vi "BatteryWarningTest_3.2V.vi"(8 "error in":errorcluster) -> (0 "error in (no error)":errorcluster, 1 "Pass/Fail":bool, 4 "Limit2":u8[](array[numeric]) format="%x", 5 "Limit1":u8[](array[numeric]) format="%x")   [LabVIEW 2009]
uses:
  <vilib>/Instr/_visa.llb/VISA Configure Serial Port (Instr).vi
  Global/Global 1.vi
panel:
  # "30"
  # "0A"
  # "0A"
  # "31"
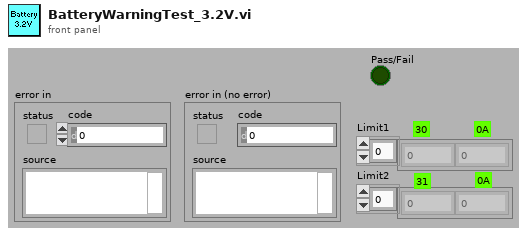
[diagram p1: front panel]
types:
  T1 = cluster{"VHEATFUSENOLOADMIN":string, "VHEATFUSELOADMAX":string, "VOVERRIDEDIODEMIN":string, "TDIFFMAX":string, "MEASFREQMAX":string, "MEASFREQMIN":string, "VOVER":string, "VMIDDLE":string, "VUNDER":string, "VNORESET":string, "VRESET":string, "WAITPING":string, "LRFID":string, "RFIDUID":string, "EXTEESIZE":string, "LCUTYPE":string, "LCUSUBTYPE":string, "TEVN":string, "BOOTVER":string, "APPVER":string, "ISLEEPMAX":string, "TSLEEP":string, "APPWAIT":string, "DBWAIT":string}
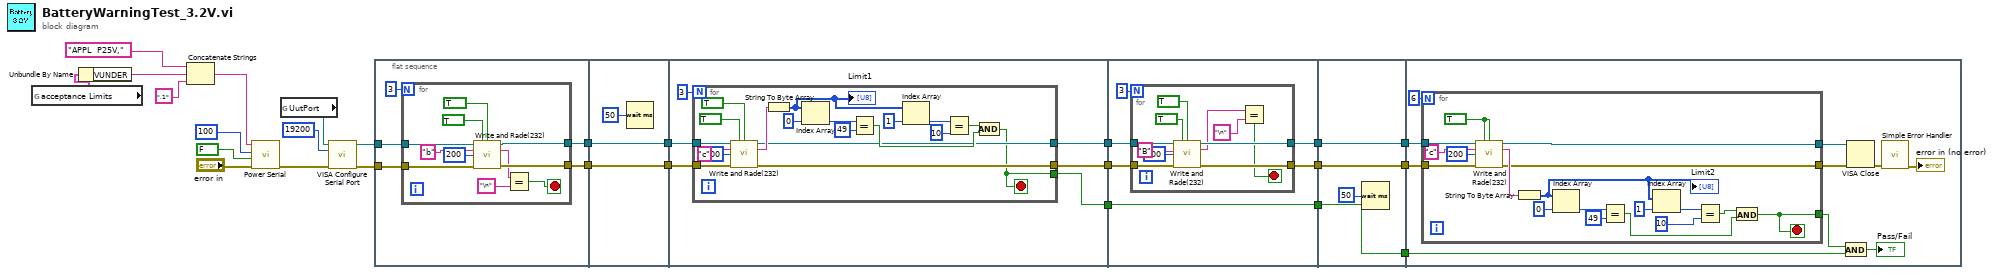
[diagram p0: block diagram]
diagram:
  n1 = global read "Global 1.vi" "acceptance Limits"() -> (w5:T1)
  n2 = Unbundle By Name(w5) -> ("VUNDER"=w4:string)
  n3 = Concatenate Strings("APPL  P25V," ("In"), w4, ",1" ("string")) -> (w1:string)
  n4 = call "Power Serial.vi"("error in (no error)"="error in", "Rd?"=FALSE, "Delay"=100, "IN"=w1) -> ("error out"=w11:errorcluster)  [unwired: 1 in, 6 out]
  n5 = global read "Global 1.vi" "UutPort"() -> (w12:refnum<visa-resource-name>)
  n6 = call-poly "VISA Configure Serial Port"("VISA resource name"=w12, "baud rate (9600)"=u32 19200, "error in (no error)"=w11) -> ("VISA resource name out"=w6:refnum<visa-resource-name>, "error out"=w7:errorcluster)  [unwired: 3 in, 8 out]
  n7 = flat-sequence {
    tunnel: [w31] -> w23
    tunnel: [w30] -> w21
    tunnel: w7 -> [w28]
    tunnel: w6 -> [w27]
    tunnel: w23 -> [w44]
    tunnel: [w44] -> w22
    tunnel: w21 -> [w43]
    tunnel: [w43] -> w20
    tunnel: [w51] -> w24
    tunnel: w22 -> [w50]
    tunnel: w20 -> [w49]
    tunnel: [w48] -> w19
    tunnel: [w47] -> w18
    tunnel: [w76] -> w25
    tunnel: w24 -> [w76]
    tunnel: w19 -> [w75]
    tunnel: w18 -> [w74]
    tunnel: [w73] -> w17
    tunnel: [w72] -> w15
    tunnel: [w90] -> w26
    tunnel: w25 -> [w90]
    tunnel: w17 -> [w89]
    tunnel: [w89] -> w16
    tunnel: w15 -> [w88]
    tunnel: [w88] -> w14
    tunnel: w26 -> [w101]
    tunnel: w16 -> [w98]
    tunnel: w14 -> [w97]
    frame #0 {
      n8 = for {
        N: 3 -> [_]
        tunnel: w28 -> [w41]
        tunnel: w27 -> [w40]
        tunnel: [w39] -> w31
        tunnel: [w38] -> w30
        stop <- w33 stop-if-true
        n9 = call "Write and Rade(232).vi"("VISA resource name in"=w40, "write"=TRUE, "read"=TRUE, "string to write"="b", "ms delay"=u32 200, "error in"=w41) -> ("VISA resource name out"=w39:refnum<visa-resource-name>, "read string"=w35:string, "error out"=w38:errorcluster)  [unwired: 2 in, 5 out]
        n10 = Equal?(x=w35, y="\n") -> (x = y?=w33:bool)
      }
    }
    frame #1 {
      n11 = Wait (ms)(milliseconds to wait=u32 50) -> ()  [unwired: 1 out]
    }
    frame #2 {
      n12 = for {
        N: 3 -> [_]
        tunnel: [w53] -> w51
        tunnel: w50 -> [w60]
        tunnel: w49 -> [w59]
        tunnel: [w55] -> w48
        tunnel: [w54] -> w47
        stop <- w53 stop-if-true
        n13 = call "Write and Rade(232).vi"("VISA resource name in"=w60, "write"=TRUE, "read"=TRUE, "string to write"="c", "ms delay"=u32 200, "error in"=w59) -> ("VISA resource name out"=w54:refnum<visa-resource-name>, "read string"=w56:string, "error out"=w55:errorcluster)  [unwired: 2 in, 5 out]
        n14 = String To Byte Array(string=w56) -> (unsigned byte array=w65:u8[])
        "Limit1" <- w65
        n15 = Index Array(array=w65, index=0) -> (element=w63:u8)
        n16 = Equal?(x=w63, y=u8 49) -> (x = y?=w70:bool)
        n17 = Index Array(array=w65, index=1) -> (element=w67:u8)
        n18 = Equal?(x=w67, y=u8 10) -> (x = y?=w69:bool)
        n19 = And(x=w69, y=w70) -> (x .and. y?=w53:bool)
      }
    }
    frame #3 {
      n20 = for {
        N: 3 -> [_]
        tunnel: w75 -> [w87]
        tunnel: w74 -> [w85]
        tunnel: [w84] -> w73
        tunnel: [w83] -> w72
        stop <- w78 stop-if-true
        n21 = call "Write and Rade(232).vi"("VISA resource name in"=w85, "write"=TRUE, "read"=TRUE, "string to write"="B", "ms delay"=u32 200, "error in"=w87) -> ("VISA resource name out"=w83:refnum<visa-resource-name>, "read string"=w80:string, "error out"=w84:errorcluster)  [unwired: 2 in, 5 out]
        n22 = Equal?(x=w80, y="\n") -> (x = y?=w78:bool)
      }
    }
    frame #4 {
      n23 = Wait (ms)(milliseconds to wait=u32 50) -> ()  [unwired: 1 out]
    }
    frame #5 {
      n24 = for {
        N: 6 -> [_]
        tunnel: [w103] -> w99
        tunnel: w98 -> [w109]
        tunnel: w97 -> [w108]
        tunnel: [w106] -> w96
        tunnel: [w105] -> w94
        stop <- w103 stop-if-true
        w104 = TRUE ("write")
        n25 = call "Write and Rade(232).vi"("VISA resource name in"=w108, "write"=w104, "read"=w104, "string to write"="c", "ms delay"=u32 200, "error in"=w109) -> ("VISA resource name out"=w105:refnum<visa-resource-name>, "read string"=w107:string, "error out"=w106:errorcluster)  [unwired: 2 in, 5 out]
        n26 = String To Byte Array(string=w107) -> (unsigned byte array=w115:u8[])
        "Limit2" <- w115
        n27 = Index Array(array=w115, index=0) -> (element=w113:u8)
        n28 = Equal?(x=w113, y=u8 49) -> (x = y?=w119:bool)
        n29 = Index Array(array=w115, index=1) -> (element=w117:u8)
        n30 = Equal?(x=w117, y=u8 10) -> (x = y?=w111:bool)
        n31 = And(x=w111, y=w119) -> (x .and. y?=w103:bool)
      }
      n32 = And(x=w99, y=w101) -> (x .and. y?=→"Pass/Fail":bool)
      n33 = VISA Close(VISA resource name=w94, error in (no error)=w96) -> (error out=w95:errorcluster)
      n34 = call <vilib>:"Simple Error Handler.vi"("error in (no error)"=w95) -> ("error out"=→"error in (no error)":errorcluster)  [unwired: 1 in, 7 out]
    }
  }
